vi "Buy Any.vi"(11 "Maximum Price":string) -> (3 "resulting prompt":string)   [LabVIEW 2020, in "Full Featured MCP Server.lvlib"]
doc: "Buys any stocks below the maximum price once."
uses:
  Full Featured MCP Server.lvlib
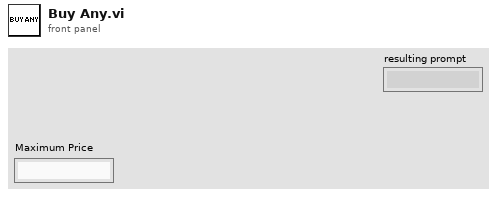
[diagram p1: front panel]
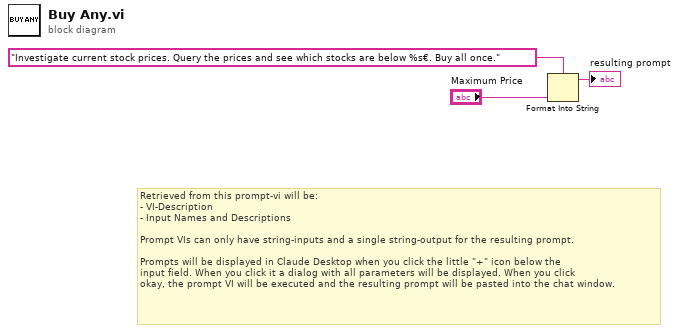
[diagram p0: block diagram]
diagram:
  # "Retrieved from this prompt-vi will be:\n- VI-Description\n- Input Names and Descriptions\n\nPrompt VIs can only have string-inputs and a single string-output for the resulting prompt.\n\nPrompts will be displayed in Claude Desktop when you click the little \"+\" icon below the \ninput field. When you click it a dialog with all parameters will be displayed. When you click\nokay, the prompt VI will be executed and the resulting prompt will be pasted into the chat window."
  n1 = Format Into String(format string="Investigate current stock prices. Query the prices and see which stocks are below %s€. Buy all once.", "Maximum Price") -> (resulting string=→"resulting prompt":string)  [unwired: 2 in, 1 out]
